vi "Launch Nested Error Reporter Actor.vi"(4 "Debug Alias":string, 6 "Open Actor Core front panel? (F)":bool, 8 "error in (no error)":errorcluster, 9 "Auto-stop? (T)":bool=TRUE, 10 "Nested Actor in":refnum<class "Error Reporter.lvclass">, 11 "Caller Actor in":refnum<class "Error Reporter.lvclass">) -> (0 "error out":errorcluster, 2 "Nested Actor's Enqueuer":refnum<class "Message Enqueuer.lvclass">, 3 "Caller Actor out":refnum<class "Error Reporter.lvclass">)   [LabVIEW 2024, in "Error Reporting Actor.lvlib" / "Error Reporter.lvlib" / "Error Reporter.lvclass"]
uses:
  Error Reporter.lvclass
  C:/Program Files (x86)/National Instruments/LabVIEW 2024/vi.lib/ActorFramework/Actor/Actor.lvclass
  <vilib>/ActorFramework/Message Enqueuer/Message Enqueuer.lvclass
  Error Reporter.lvclass/Error Reporter.ctl
  <vilib>/ActorFramework/Actor/Actor.lvclass
  C:/Users/uspoaotto/OneDrive - Oregon Tool/Desktop/working copies/errorReportingActor/src/Error Reporting Actor/Error Reporter/Error Reporter/Error Reporter.lvclass
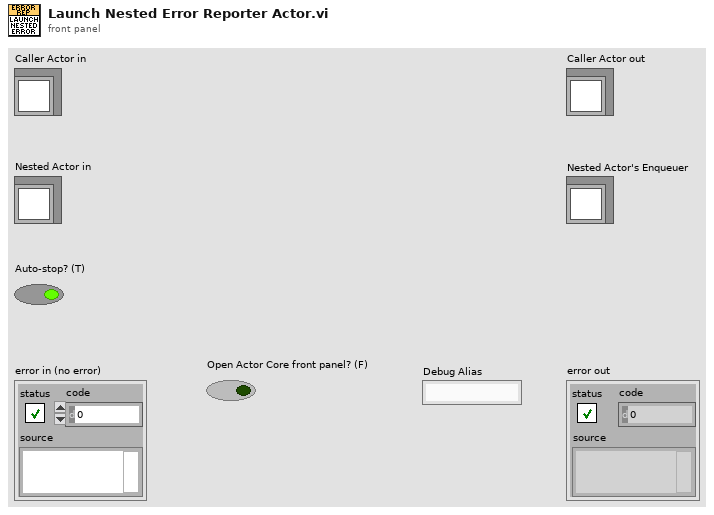
[diagram p1: front panel]
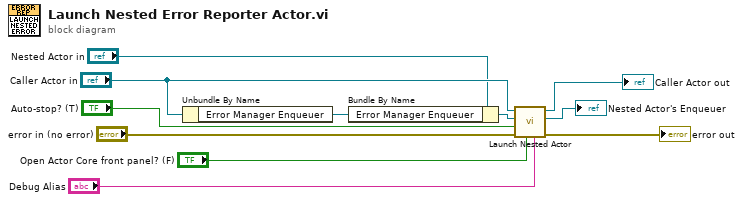
[diagram p0: block diagram]
diagram:
  n1 = Unbundle By Name("Caller Actor in") -> ("Error Manager Enqueuer"=w5:refnum<class "Message Enqueuer.lvclass">)
  n2 = Bundle By Name(cluster="Nested Actor in", "Error Manager Enqueuer"=w5) -> (w4:refnum<class "Error Reporter.lvclass">)
  n3 = call <vilib>:"Launch Nested Actor.vi"("Debug Alias"="Debug Alias", "Open Actor Core front panel? (F)"="Open Actor Core front panel? (F)", "error in (no error)"="error in (no error)", "Auto-stop? (T)"="Auto-stop? (T)", "Nested Actor"=w4, "Caller Actor in"="Caller Actor in") -> ("error out"=→"error out":errorcluster, "Nested Actor's Enqueuer"=→"Nested Actor's Enqueuer":refnum<class "Message Enqueuer.lvclass">, "Caller Actor out"=→"Caller Actor out":refnum<class "Error Reporter.lvclass">)  [unwired: 3 in]
